vi "Init MLBox.vi"(8 "error in (no error)":errorcluster, 11 "Table View in":refnum<class "Table View.lvclass">) -> (0 "error out":errorcluster, 3 "Table View out":refnum<class "Table View.lvclass">)   [LabVIEW 2020, in "[V]Table View.lvlib" / "Table View.lvclass"]
uses:
  Table View.lvclass
  <vilib>/HUASUI/MulListBox/Type Definitions/Autosize Mode.ctl
  Table View.lvclass/Table View.ctl
  <vilib>/HUASUI/MulListBox/MListBox.lvclass
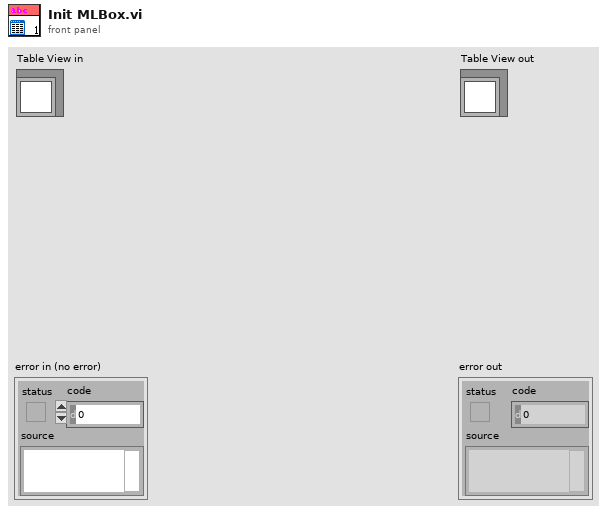
[diagram p1: front panel]
types:
  T1 = typedef "Autosize Mode.ctl" = enum16{"Header", "All Cells"}
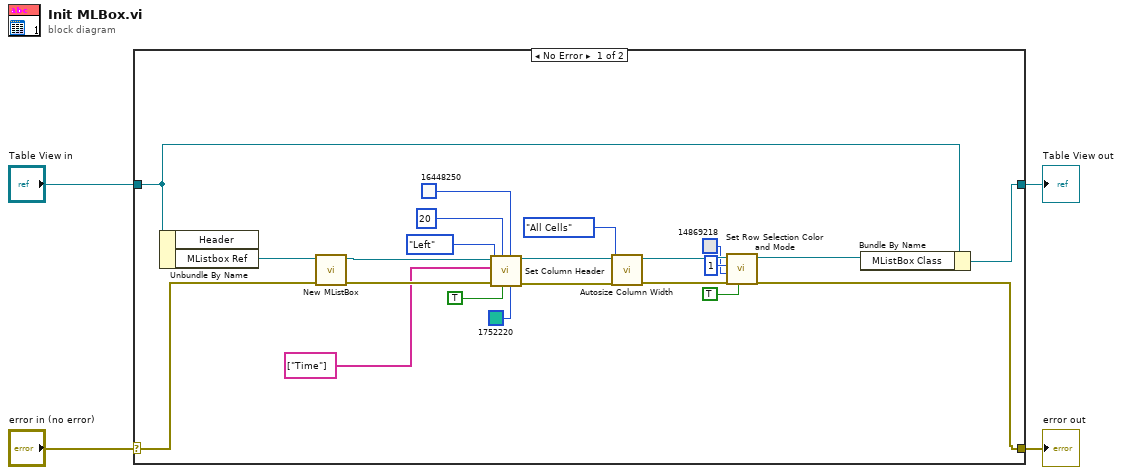
[diagram p0: block diagram]
diagram:
  n1 = case shown="No Error" "error in (no error)" {
    selector: "error in (no error)" -> [w16 w27]
    tunnel: [w11 w27] -> w3
    tunnel: [w17 w26] -> w1
    tunnel: "Table View in" -> [w18 w26]
    frame No Error {
      n2 = Unbundle By Name(w18) -> ("MListbox Ref"=w25:refnum<vi>)  [unwired: 1 out]
      n3 = call <vilib>:"New MListBox.vi"("error in (no error)"=w16, "MListbox Ref"=w25) -> ("error out"=w15:errorcluster, "Multicolumn ListBox out"=w19:refnum<class "MListBox.lvclass">)  [unwired: 8 in]
      n4 = call <vilib>:"Set Column Header.vi"("BackColor"=u32 1752220 ("Header Backcolor"), "Font Color"=u32 16448250, "Active Cell:Cell Font:Bold"=TRUE, "Font:Size"=u32 20, "error in (no error)"=w15, "Justification"=enum16{"Left", "Center", "Right"}."Left", "Column Headers"=string[] ["Time"], "Multicolumn ListBox in"=w19) -> ("error out"=w12:errorcluster, "Multicolumn ListBox out"=w13:refnum<class "MListBox.lvclass">)  [unwired: 2 in]
      n5 = call <vilib>:"Autosize Column Width.vi"("error in (no error)"=w12, "Autosize Mode"=Autosize_Mode."All Cells", "Multicolumn ListBox in"=w13) -> ("error out"=w11:errorcluster, "Multicolumn ListBox out"=w9:refnum<class "MListBox.lvclass">)  [unwired: 7 in]
      n6 = call <vilib>:"Set Row Selection Color and Mode.vi"("Select Entire Rows"=TRUE, "Selected Color"=u32 14869218, "Selection Mode"=1, "Multicolumn ListBox in"=w9) -> ("Multicolumn ListBox out"=w8:refnum<class "MListBox.lvclass">)  [unwired: 6 in, 1 out]
      n7 = Bundle By Name(cluster=w18, "MListBox Class"=w8) -> (w17:refnum<class "Table View.lvclass">)
    }
    frame Error {
    }
  }
  "error out" <- w3
  "Table View out" <- w1
